vi "GenerateFakeSignal.vi"(9 "SecondaryDataVIRef":refnum<vi>, 10 "Array":i32[](array[numeric])) -> (2 "simulated signal":i32[](array[numeric]))   [LabVIEW 2013, in "GenericDAQ.lvlib"]
uses:
  GenericDAQ.lvlib
  <vilib>/gmath/SpecialFunctions.llb/Error Function.vi
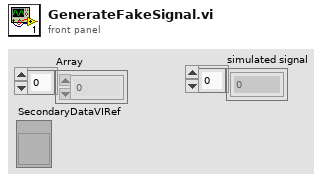
[diagram p1: front panel]
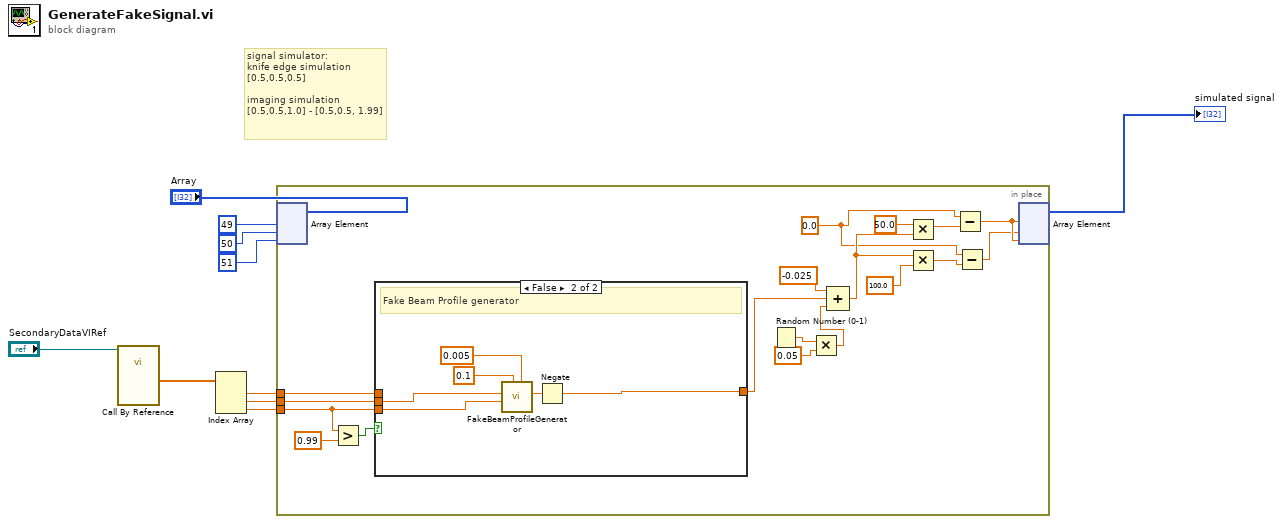
[diagram p0: block diagram]
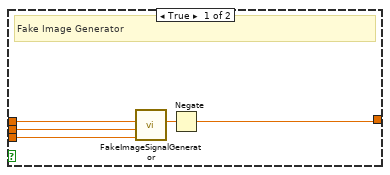
[diagram p2: hidden frame]
diagram:
  # "signal simulator:\nknife edge simulation\n[0.5,0.5,0.5]\n\nimaging simulation\n[0.5,0.5,1.0] - [0.5,0.5, 1.99]"
  n1 = call-by-ref "?"(reference="SecondaryDataVIRef") -> ("SecondaryData"=w7:dbl[])  [unwired: 12 in, 2 out]
  n2 = Index Array(array=w7) -> (element #1=w6:dbl, element #2=w5:dbl, element #3=w4:dbl)  [unwired: 3 in]
  n3 = in-place {
    in-place-border: w6 -> [w16]
    in-place-border: w5 -> [w15]
    in-place-border: w4 -> [w13]
    w11 = 0.0
    n4 = in-place-array #1("Array", 49, 50, 51) -> ()  [unwired: 3 out]
    n5 = Greater?(x=w13, y=0.99) -> (0:w14:bool)
    n6 = case shown="False" w14 {
      tunnel: [w33 w39] -> w25
      tunnel: w16 -> [w31 _]
      tunnel: w15 -> [w30 w34]
      tunnel: w13 -> [w29 w35]
      frame True {
        # "Fake Image Generator"
        n7 = call "FakeImageSignalGenerator.vi"("Z"=w29, "Y"=w30, "X"=w31) -> ("E"=w32:dbl)  [unwired: 8 in]
        n8 = Negate(x=w32) -> (-x=w33:dbl)
      }
      frame False {
        # "Fake Beam Profile generator"
        n9 = call "FakeBeamProfileGenerator.vi"("w_0"=0.005, "Z_0"=0.1, "Z"=w35, "Y"=w34) -> ("E"=w38:dbl)  [unwired: 7 in]
        n10 = Negate(x=w38) -> (-x=w39:dbl)
      }
    }
    n11 = Random Number (0-1)() -> (number: 0 to 1=w26:dbl)
    n12 = Multiply(x=w26, y=0.05) -> (x*y=w28:dbl)
    n13 = Compound Arithmetic op=ADD(-0.025 ("value"), w25, w28) -> (w24:dbl)
    n14 = Multiply(x=50.0, y=w24) -> (x*y=w21:dbl)
    n15 = Multiply(x=w24, y=100.0 ("x*y")) -> (x*y=w18:dbl)
    n16 = Subtract(x=w11, y=w21) -> (x-y=w20:dbl)
    n17 = Subtract(x=w11, y=w18) -> (x-y=w19:dbl)
    n18 = in-place-array #1(w20, w19, w20) -> (→"simulated signal":i32[])  [unwired: 3 out]
  }
